vi "Output_Trav_Pos.vi"(4 "Positions to Output":T1) -> (1 "error out":errorcluster)   [LabVIEW 2011]
uses:
  Controls/Positions.ctl
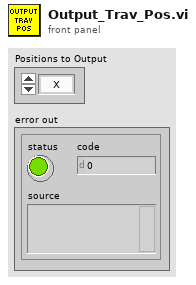
[diagram p1: front panel]
types:
  T1 = typedef "Positions.ctl" = enum16{"X", "Y", "Z", "XY", "XZ", "YZ", "XYZ"}
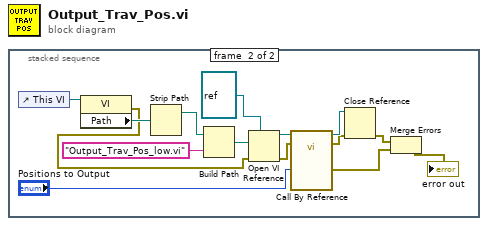
[diagram p0: block diagram]
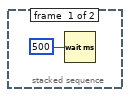
[diagram p2: hidden frame]
diagram:
  n1 = stacked-sequence {
    frame #0 {
      n2 = Wait (ms)(milliseconds to wait=u32 500) -> ()  [unwired: 1 out]
    }
    frame #1 {
      n3 = control-ref of="This VI"() -> (w16:refnum<vi>)
      n4 = property class="VI"(reference=w16) -> (error out=w7:errorcluster, "Path"=w14:path)  [unwired: 1 in, 1 out]
      n5 = Strip Path(path=w14) -> (stripped path=w13:path)  [unwired: 1 out]
      n6 = Build Path(base path=w13, name or relative path="Output_Trav_Pos_low.vi") -> (appended path=w11:path)
      n7 = Open VI Reference(type specifier VI Refnum (for type only)=refnum<vi> refnum, vi path=w11, error in (no error)=w7) -> (vi reference=w10:refnum<vi>, error out=w6:errorcluster)  [unwired: 3 in]
      n8 = call-by-ref "?"(reference=w10, error in=w6, "Positions to Output"="Positions to Output") -> (reference out=w8:refnum<vi>, error out=w5:errorcluster, 1:"error out"=w4:errorcluster)  [unwired: 4 in]
      n9 = Close Reference(reference=w8, error in (no error)=w5) -> (error out=w3:errorcluster)
      n10 = Merge Errors(w3, w4) -> (→"error out":errorcluster)
    }
  }
